vi "Load App.vi"(8 "错误输入（无错误）":errorcluster, 11 "通知器":refnum<notifier>) -> (0 "error out":errorcluster caption="错误输出")   [LabVIEW 2017, in "TPP demo V2.lvlib" / "TPP demo V2.lvclass"]
uses:
  TPP demo V2.lvclass
  E:/Program Files (x86)/National Instruments/LabVIEW 2017/vi.lib/ActorFramework/Actor/Actor.lvclass
  <vilib>/ActorFramework/Actor/Actor.lvclass
panel:
  in  "TPP demo V2.lvlib:TPP demo V2.lvclass":refnum<class "TPP demo V2.lvclass">
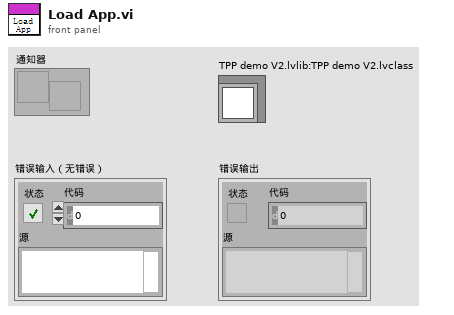
[diagram p1: front panel]
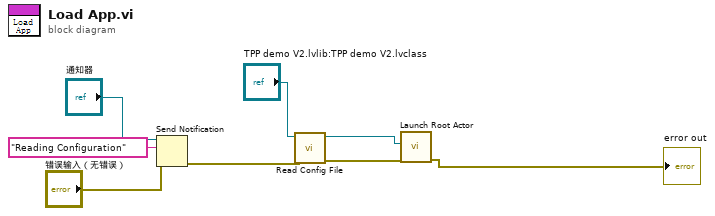
[diagram p0: block diagram]
diagram:
  n1 = Send Notification(notification="Reading Configuration" ("通知"), notifier="通知器", error in (no error)="错误输入（无错误）") -> (error out=w5:errorcluster)  [unwired: 1 out]
  n2 = call-dynamic "Read Config File.vi"("error in (no error)"=w5, "TPP demo V2 输入"="TPP demo V2.lvlib:TPP demo V2.lvclass") -> ("error out"=w4:errorcluster, "TPP demo V2 输出"=w3:refnum<class "TPP demo V2.lvclass">)  [unwired: 8 in]
  n3 = call <vilib>:"Launch Root Actor.vi"("error in (no error)"=w4, "Actor"=w3) -> ("error out"=→"error out":errorcluster)  [unwired: 8 in, 1 out]
